vi "Copy Test.vi"() -> ()   [LabVIEW 2020, in "Test Executive.lvlib"]
uses:
  <vilib>/gpm_packages/@cs/test-executive/Source/Test Executive/Test Executive.lvlib
  <vilib>/gpm_packages/@cs/test-executive/Source/Test Executive/TestExecutive/Test Executive.lvclass
  C:/Program Files/National Instruments/LabVIEW 2020/vi.lib/gpm_packages/@cs/test-executive/Source/Test Executive/ITestExecutive/ITest Executive.lvclass
  <vilib>/gpm_packages/@cs/test-executive/Source/Test Executive/Executioner/Executioner.lvclass
  <vilib>/gpm_packages/@cs/run-time-assertions/Source/Assert Equal/Assert Equal.lvclass
  C:/Program Files/National Instruments/LabVIEW 2020/vi.lib/gpm_packages/@cs/run-time-assertions/Source/Assert/Assert.lvclass
  <vilib>/gpm_packages/@cs/run-time-assertions/Source/Assert Greater/Assert Greater.lvclass
  <vilib>/gpm_packages/@cs/run-time-assertions/Source/Assert Less/Assert Less.lvclass
  e1a8998e-4afa-4658-809d-ffab1fdc1dd3.vi
  2b1bbdfa-28ea-4975-b67d-55fb8ecea142.vi
  38d44331-03b6-4e0e-b502-f580cf716a25.vi
  13797e50-8b76-425b-83b2-76a457203fcb.vi
  82e98dc6-0186-4ac9-b806-f29624e46a62.vi
  c7986c9b-765c-4e35-9bdb-656a1762b2cf.vi
  5b298818-1d60-4780-a578-24e6083b1334.vi
  313207bc-dc89-4460-a504-7f065ccd0a73.vi
  3f58f81d-24f4-4b38-8029-ea7739ca710f.vi
  4ea763fe-e262-4f1b-8a79-0ca79b847688.vi
  6a21370e-3cef-4ac3-8829-bf63652873b0.vi
  103630d6-5241-4d15-b3ff-21d61f4a4c4c.vi
  36607b50-8362-4d71-bcc6-c0885ffd9225.vi
  6c5806c5-2cdd-491e-b3b5-fcdc1241d2ce.vi
  b891e3ce-f0ac-467a-8f2d-10a6ff9ae12a.vi
  <vilib>/Utility/error.llb/Error Cluster From Error Code.vi
  <vilib>/gpm_packages/@cs/test-executive/Source/Test Executive/ITestExecutive/ITest Executive.lvclass
  <vilib>/gpm_packages/@cs/test-executive/Source/Test Executive/TestExecutive Ref/TestExecutive Ref.lvclass
panel:
  out "X Var post":string[](array[string])
  out "Y Var post":string[](array[string])
  out "Y Var pre":string[](array[string])
  out "X Var pre":string[](array[string])
  in  "Tree Post Copy":string(tree)
  in  "Tree":string(tree)
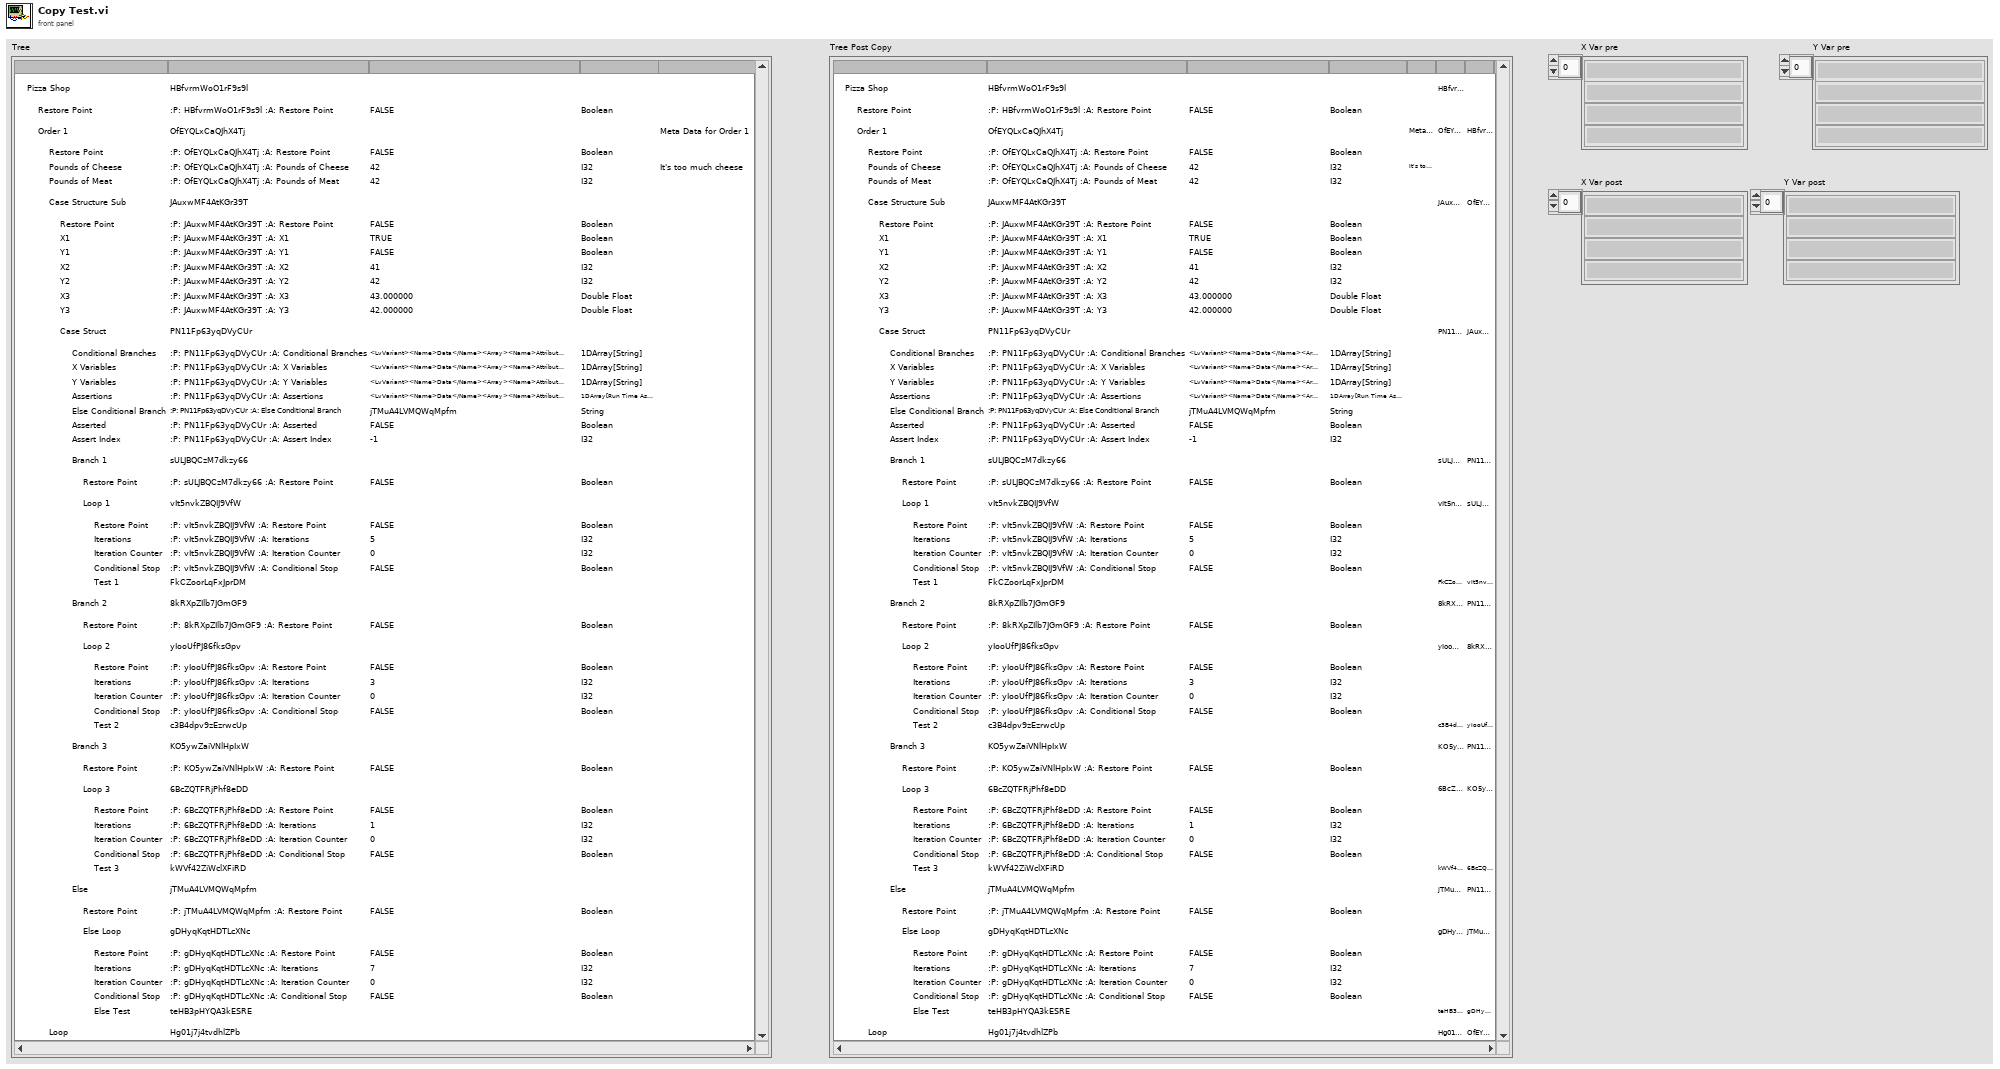
[diagram p1: front panel]
types:
  T1 = cluster{"Left Cell String":string, "Child Text":string[], "Child Tag":string, "Item Indent":i32, "Child Only?":bool, "Glyph Index":i32}[]
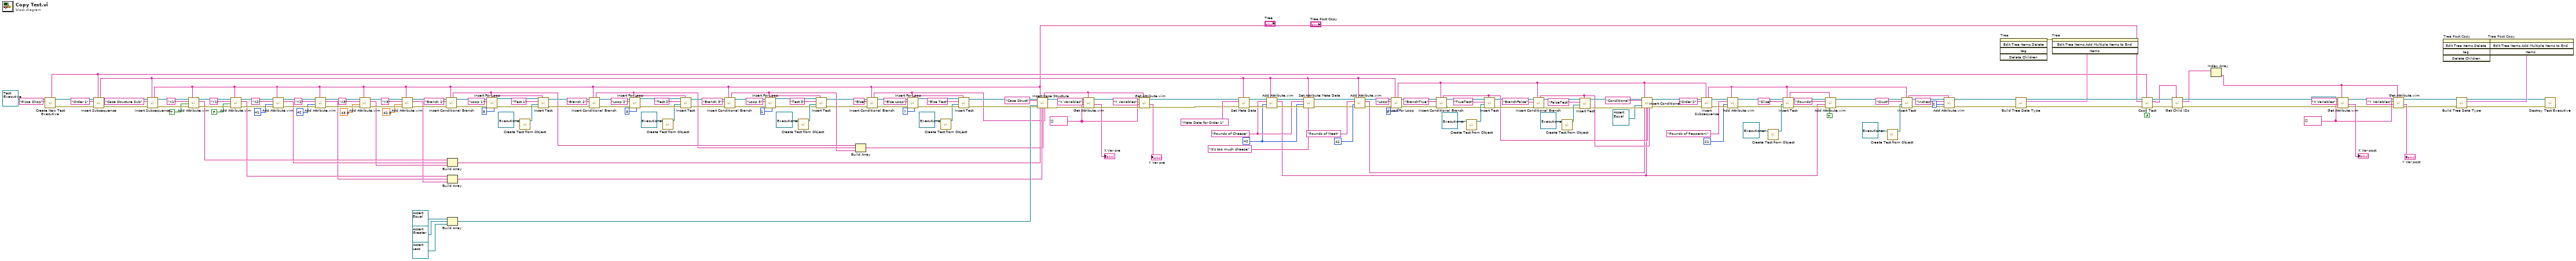
[diagram p0: block diagram]
diagram:
  w15 = string[] []
  w21 = string[] []
  w134 = 42
  w135 = "Pounds of Cheese" ("Attribute Name")
  n1 = call <vilib>:"Create New Test Executive.vi"("Name"="Pizza Shop", "Test Executive"=refnum<class "Test Executive.lvclass"> refnum ("Test Executive.lvlib:Test Executive.lvclass")) -> ("error out"=w208:errorcluster, "Test Executive Ref"=w209:refnum<data-value>, "Test Executive ID out"=w133:string)  [unwired: 7 in]
  n2 = call <vilib>:"Insert Subsequence.vi"("Parent ID"=w133, "error in (no error)"=w208, "Name"="Order 1", "Test Executive Ref"=w209) -> ("error out"=w30:errorcluster, "Test Executive Ref out"=w31:refnum<data-value>, "Unique ID out"=w32:string)  [unwired: 4 in, 1 out]
  n3 = call <vilib>:"Insert Subsequence.vi"("Parent ID"=w32, "error in (no error)"=w30, "Name"="Case Structure Sub", "Test Executive Ref"=w31) -> ("error out"=w127:errorcluster, "Test Executive Ref out"=w128:refnum<data-value>, "Unique ID out"=w8:string)  [unwired: 4 in, 1 out]
  n4 = call "Add Attribute.vim"("ID"=w8, "error in (no error)"=w127, "Attribute"=TRUE, "Attribute Name"="X1", "Test Executive Ref"=w128) -> ("error out"=w121:errorcluster, "Attribute ID out"=w61:string, "Test Executive Ref out"=w122:refnum<data-value>)  [unwired: 3 in, 1 out]
  n5 = call "Add Attribute.vim"("ID"=w8, "error in (no error)"=w121, "Attribute"=FALSE, "Attribute Name"="Y1", "Test Executive Ref"=w122) -> ("error out"=w113:errorcluster, "Attribute ID out"=w58:string, "Test Executive Ref out"=w114:refnum<data-value>)  [unwired: 3 in, 1 out]
  n6 = call "Add Attribute.vim"("ID"=w8, "error in (no error)"=w113, "Attribute"=41, "Attribute Name"="X2", "Test Executive Ref"=w114) -> ("error out"=w120:errorcluster, "Attribute ID out"=w60:string, "Test Executive Ref out"=w119:refnum<data-value>)  [unwired: 3 in, 1 out]
  n7 = call "Add Attribute.vim"("ID"=w8, "error in (no error)"=w120, "Attribute"=42, "Attribute Name"="Y2", "Test Executive Ref"=w119) -> ("error out"=w105:errorcluster, "Attribute ID out"=w57:string, "Test Executive Ref out"=w106:refnum<data-value>)  [unwired: 3 in, 1 out]
  n8 = call "Add Attribute.vim"("ID"=w8, "error in (no error)"=w105, "Attribute"=43.0, "Attribute Name"="X3", "Test Executive Ref"=w106) -> ("error out"=w107:errorcluster, "Attribute ID out"=w59:string, "Test Executive Ref out"=w108:refnum<data-value>)  [unwired: 3 in, 1 out]
  n9 = call "Add Attribute.vim"("ID"=w8, "error in (no error)"=w107, "Attribute"=42.0, "Attribute Name"="Y3", "Test Executive Ref"=w108) -> ("error out"=w102:errorcluster, "Attribute ID out"=w56:string, "Test Executive Ref out"=w104:refnum<data-value>)  [unwired: 3 in, 1 out]
  n10 = call <vilib>:"Insert Conditional Branch.vi"("Parent ID"=w8, "error in (no error)"=w102, "Name"="Branch 1", "Test Executive Ref"=w104) -> ("error out"=w98:errorcluster, "Test Executive Ref out"=w100:refnum<data-value>, "Unique ID out"=w53:string)  [unwired: 4 in, 1 out]
  n11 = Build Array(w61, w60, w59) -> (w55:string[])
  n12 = Build Array(w58, w57, w56) -> (w54:string[])
  n13 = Build Array(refnum<class "Assert Equal.lvclass"> refnum ("Run Time Assertions.lvlib:Assert Equal.lvclass"), refnum<class "Assert Greater.lvclass"> refnum ("Run Time Assertions.lvlib:Assert Greater.lvclass"), refnum<class "Assert Less.lvclass"> refnum ("Run Time Assertions.lvlib:Assert Less.lvclass")) -> (w62:refnum<class "Assert.lvclass">[])
  n14 = call <vilib>:"Insert For Loop.vi"("Loop Iterations"=5, "Parent ID"=w53, "error in (no error)"=w98, "Name"="Loop 1", "Test Executive Ref"=w100) -> ("error out"=w94:errorcluster, "Test Executive Ref out"=w93:refnum<data-value>, "Unique ID out"=w92:string)  [unwired: 3 in, 1 out]
  n15 = call <vilib>:"Create Test from Object.vi"("Test"=refnum<class "Executioner.lvclass"> refnum ("Test Executive.lvlib:Executioner.lvclass")) -> ("Test"=w95:refnum<class "Executioner.lvclass">)  [unwired: 10 in]
  n16 = call <vilib>:"Insert Test.vi"("Parent ID"=w92, "error in (no error)"=w94, "Test"=w95, "Name"="Test 1", "Test Executive Ref"=w93) -> ("error out"=w79:errorcluster, "Test Executive Ref out"=w80:refnum<data-value>)  [unwired: 3 in, 2 out]
  n17 = call <vilib>:"Insert Conditional Branch.vi"("Parent ID"=w8, "error in (no error)"=w79, "Name"="Branch 2", "Test Executive Ref"=w80) -> ("error out"=w85:errorcluster, "Test Executive Ref out"=w83:refnum<data-value>, "Unique ID out"=w52:string)  [unwired: 4 in, 1 out]
  n18 = call <vilib>:"Insert For Loop.vi"("Loop Iterations"=3, "Parent ID"=w52, "error in (no error)"=w85, "Name"="Loop 2", "Test Executive Ref"=w83) -> ("error out"=w89:errorcluster, "Test Executive Ref out"=w90:refnum<data-value>, "Unique ID out"=w91:string)  [unwired: 3 in, 1 out]
  n19 = call <vilib>:"Create Test from Object.vi"("Test"=refnum<class "Executioner.lvclass"> refnum ("Test Executive.lvlib:Executioner.lvclass")) -> ("Test"=w88:refnum<class "Executioner.lvclass">)  [unwired: 10 in]
  n20 = call <vilib>:"Insert Test.vi"("Parent ID"=w91, "error in (no error)"=w89, "Test"=w88, "Name"="Test 2", "Test Executive Ref"=w90) -> ("error out"=w66:errorcluster, "Test Executive Ref out"=w67:refnum<data-value>)  [unwired: 3 in, 2 out]
  n21 = call <vilib>:"Insert Conditional Branch.vi"("Parent ID"=w8, "error in (no error)"=w66, "Name"="Branch 3", "Test Executive Ref"=w67) -> ("error out"=w74:errorcluster, "Test Executive Ref out"=w76:refnum<data-value>, "Unique ID out"=w51:string)  [unwired: 4 in, 1 out]
  n22 = call <vilib>:"Insert For Loop.vi"("Loop Iterations"=1, "Parent ID"=w51, "error in (no error)"=w74, "Name"="Loop 3", "Test Executive Ref"=w76) -> ("error out"=w70:errorcluster, "Test Executive Ref out"=w69:refnum<data-value>, "Unique ID out"=w68:string)  [unwired: 3 in, 1 out]
  n23 = call <vilib>:"Create Test from Object.vi"("Test"=refnum<class "Executioner.lvclass"> refnum ("Test Executive.lvlib:Executioner.lvclass")) -> ("Test"=w71:refnum<class "Executioner.lvclass">)  [unwired: 10 in]
  n24 = call <vilib>:"Insert Test.vi"("Parent ID"=w68, "error in (no error)"=w70, "Test"=w71, "Name"="Test 3", "Test Executive Ref"=w69) -> ("error out"=w37:errorcluster, "Test Executive Ref out"=w38:refnum<data-value>)  [unwired: 3 in, 2 out]
  n25 = Build Array(w53, w52, w51) -> (w50:string[])
  n26 = call <vilib>:"Insert Conditional Branch.vi"("Parent ID"=w8, "error in (no error)"=w37, "Name"="Else", "Test Executive Ref"=w38) -> ("error out"=w43:errorcluster, "Test Executive Ref out"=w41:refnum<data-value>, "Unique ID out"=w34:string)  [unwired: 4 in, 1 out]
  n27 = call <vilib>:"Insert For Loop.vi"("Loop Iterations"=7, "Parent ID"=w34, "error in (no error)"=w43, "Name"="Else Loop", "Test Executive Ref"=w41) -> ("error out"=w47:errorcluster, "Test Executive Ref out"=w48:refnum<data-value>, "Unique ID out"=w49:string)  [unwired: 3 in, 1 out]
  n28 = call <vilib>:"Create Test from Object.vi"("Test"=refnum<class "Executioner.lvclass"> refnum ("Test Executive.lvlib:Executioner.lvclass")) -> ("Test"=w46:refnum<class "Executioner.lvclass">)  [unwired: 10 in]
  n29 = call <vilib>:"Insert Test.vi"("Parent ID"=w49, "error in (no error)"=w47, "Test"=w46, "Name"="Else Test", "Test Executive Ref"=w48) -> ("error out"=w36:errorcluster, "Test Executive Ref out"=w35:refnum<data-value>)  [unwired: 3 in, 2 out]
  n30 = call <vilib>:"Insert Case Structure.vi"("Test Executive Ref"=w35, "Name"="Case Struct", "Assertions"=w62, "error in (no error)"=w36, "Parent ID"=w8, "X Variables"=w55, "Y Variables"=w54, "Conditional Branches"=w50, "\"Else\" Conditional Branch"=w34) -> ("Unique ID out"=w18:string, "Test Executive Ref out"=w29:refnum<data-value>, "error out"=w28:errorcluster)  [unwired: 7 in, 1 out]
  n31 = call "Get Attribute.vim"("ID"=w18, "error in (no error)"=w28, "Type"=w21, "Attribute Name"="X Variables", "Test Executive Ref"=w29) -> ("error out"=w23:errorcluster, "Attribute"=→"X Var pre":string[], "Test Executive Ref out"=w25:refnum<data-value>)  [unwired: 2 in, 2 out]
  n32 = call "Get Attribute.vim"("ID"=w18, "error in (no error)"=w23, "Type"=w21, "Attribute Name"="Y Variables", "Test Executive Ref"=w25) -> ("error out"=w22:errorcluster, "Attribute"=→"Y Var pre":string[], "Test Executive Ref out"=w24:refnum<data-value>)  [unwired: 2 in, 2 out]
  n33 = call <vilib>:"Set Meta Data.vi"("Unique ID"=w32, "error in (no error)"=w22, "Meta Data"="Meta Data for Order 1", "Test Executive Ref"=w24) -> ("error out"=w141:errorcluster, "Test Executive Ref out"=w142:refnum<data-value>)  [unwired: 6 in]
  n34 = call "Add Attribute.vim"("ID"=w32, "error in (no error)"=w141, "Attribute"=w134, "Attribute Name"=w135, "Test Executive Ref"=w142) -> ("error out"=w137:errorcluster, "Attribute ID out"=w130:string, "Test Executive Ref out"=w139:refnum<data-value>)  [unwired: 3 in, 1 out]
  n35 = call <vilib>:"Set Attribute Meta Data.vi"("Meta Data"="It's too much cheese", "Unique ID"=w32, "error in (no error)"=w137, "Attribute Type"=w134, "Attribute Name"=w135, "Test Executive Ref"=w139) -> ("error out"=w136:errorcluster, "Test Executive Ref out"=w138:refnum<data-value>)  [unwired: 3 in, 1 out]
  n36 = call "Add Attribute.vim"("ID"=w32, "error in (no error)"=w136, "Attribute"=42, "Attribute Name"="Pounds of Meat", "Test Executive Ref"=w138) -> ("error out"=w146:errorcluster, "Attribute ID out"=w143:string, "Test Executive Ref out"=w147:refnum<data-value>)  [unwired: 3 in, 1 out]
  n37 = call <vilib>:"Insert For Loop.vi"("Loop Iterations"=5, "Parent ID"=w32, "error in (no error)"=w146, "Name"="Loop", "Test Executive Ref"=w147) -> ("error out"=w152:errorcluster, "Test Executive Ref out"=w154:refnum<data-value>, "Unique ID out"=w150:string)  [unwired: 3 in, 1 out]
  n38 = call <vilib>:"Insert Conditional Branch.vi"("Parent ID"=w150, "error in (no error)"=w152, "Name"="BranchTrue", "Test Executive Ref"=w154) -> ("error out"=w168:errorcluster, "Test Executive Ref out"=w167:refnum<data-value>, "Unique ID out"=w149:string)  [unwired: 4 in, 1 out]
  n39 = call <vilib>:"Create Test from Object.vi"("Test"=refnum<class "Executioner.lvclass"> refnum ("Test Executive.lvlib:Executioner.lvclass")) -> ("Test"=w169:refnum<class "Executioner.lvclass">)  [unwired: 10 in]
  n40 = call <vilib>:"Insert Test.vi"("Parent ID"=w149, "error in (no error)"=w168, "Test"=w169, "Name"="TrueTest", "Test Executive Ref"=w167) -> ("error out"=w161:errorcluster, "Test Executive Ref out"=w160:refnum<data-value>)  [unwired: 3 in, 2 out]
  n41 = call <vilib>:"Insert Conditional Branch.vi"("Parent ID"=w150, "error in (no error)"=w161, "Name"="BranchFalse", "Test Executive Ref"=w160) -> ("error out"=w163:errorcluster, "Test Executive Ref out"=w162:refnum<data-value>, "Unique ID out"=w148:string)  [unwired: 4 in, 1 out]
  n42 = call <vilib>:"Create Test from Object.vi"("Test"=refnum<class "Executioner.lvclass"> refnum ("Test Executive.lvlib:Executioner.lvclass")) -> ("Test"=w164:refnum<class "Executioner.lvclass">)  [unwired: 10 in]
  n43 = call <vilib>:"Insert Test.vi"("Parent ID"=w148, "error in (no error)"=w163, "Test"=w164, "Name"="FalseTest", "Test Executive Ref"=w162) -> ("error out"=w158:errorcluster, "Test Executive Ref out"=w157:refnum<data-value>)  [unwired: 3 in, 2 out]
  n44 = call <vilib>:"Insert Conditional.vi"("Test Executive Ref"=w157, "Name"="Conditional", "Assertion"=refnum<class "Assert Equal.lvclass"> refnum ("Run Time Assertions.lvlib:Assert Equal.lvclass"), "error in (no error)"=w158, "Parent ID"=w150, "Variable X"=w143, "Variable Y"=w130, "Passing Executive"=w149, "Failing Executive"=w148) -> ("Test Executive Ref out"=w153:refnum<data-value>, "error out"=w151:errorcluster)  [unwired: 7 in, 2 out]
  n45 = call <vilib>:"Insert Subsequence.vi"("Parent ID"=w150, "error in (no error)"=w151, "Name"="Order 2", "Test Executive Ref"=w153) -> ("error out"=w206:errorcluster, "Test Executive Ref out"=w205:refnum<data-value>, "Unique ID out"=w174:string)  [unwired: 4 in, 1 out]
  n46 = call "Add Attribute.vim"("ID"=w174, "error in (no error)"=w206, "Attribute"=21, "Attribute Name"="Pounds of Pepperoni", "Test Executive Ref"=w205) -> ("error out"=w193:errorcluster, "Test Executive Ref out"=w194:refnum<data-value>)  [unwired: 3 in, 2 out]
  n47 = call <vilib>:"Create Test from Object.vi"("Test"=refnum<class "Executioner.lvclass"> refnum ("Test Executive.lvlib:Executioner.lvclass")) -> ("Test"=w195:refnum<class "Executioner.lvclass">)  [unwired: 10 in]
  n48 = call <vilib>:"Insert Test.vi"("Parent ID"=w174, "error in (no error)"=w193, "Test"=w195, "Name"="Slice", "Test Executive Ref"=w194) -> ("error out"=w197:errorcluster, "Test Executive Ref out"=w200:refnum<data-value>, "Unique ID out"=w199:string)  [unwired: 3 in, 1 out]
  n49 = call "Add Attribute.vim"("Pointer?"=TRUE, "ID"=w199, "error in (no error)"=w197, "Attribute"=w130, "Attribute Name"="Pounds", "Test Executive Ref"=w200) -> ("error out"=w176:errorcluster, "Test Executive Ref out"=w178:refnum<data-value>)  [unwired: 2 in, 2 out]
  n50 = call <vilib>:"Create Test from Object.vi"("Test"=refnum<class "Executioner.lvclass"> refnum ("Test Executive.lvlib:Executioner.lvclass")) -> ("Test"=w185:refnum<class "Executioner.lvclass">)  [unwired: 10 in]
  n51 = call <vilib>:"Insert Test.vi"("Parent ID"=w174, "error in (no error)"=w176, "Test"=w185, "Name"="Crust", "Test Executive Ref"=w178) -> ("error out"=w183:errorcluster, "Test Executive Ref out"=w180:refnum<data-value>, "Unique ID out"=w173:string)  [unwired: 3 in, 1 out]
  n52 = call "Add Attribute.vim"("ID"=w173, "error in (no error)"=w183, "Attribute"=2, "Attribute Name"="Inches", "Test Executive Ref"=w180) -> ("error out"=w175:errorcluster, "Test Executive Ref out"=w177:refnum<data-value>)  [unwired: 3 in, 2 out]
  n53 = invoke on="Tree" class="Tree (strict)" method="Edit Tree Items.Delete"() -> (error out=w186:errorcluster)  [unwired: 5 in, 4 out]
  n54 = call <vilib>:"Build Tree Data Type.vi"("error in (no error)"=w175, "Test Executive Ref"=w177) -> ("error out"=w188:errorcluster, "Tree Data"=w187:T1, "Test Executive Ref out"=w189:refnum<data-value>)  [unwired: 7 in]
  n55 = invoke on="Tree" class="Tree (strict)" method="Edit Tree Items.Add Multiple Items to End"(error in=w186, "Items"=w187) -> ()  [unwired: 2 in, 4 out]
  n56 = call <vilib>:"Copy Test.vi"("Move?"=FALSE, "New Parent ID"=w133, "error in (no error)"=w188, "Test ID"=w8, "Test Executive Ref"=w189) -> ("error out"=w6:errorcluster, "Test ID out"=w2:string, "Test Executive Ref out"=w7:refnum<data-value>)  [unwired: 4 in]
  n57 = call <vilib>:"Get Child IDs.vi"("Unique ID"=w2, "error in (no error)"=w6, "Test Executive Ref"=w7) -> ("error out"=w4:errorcluster, "Child IDs"=w3:string[], "Test Executive Ref out"=w5:refnum<data-value>)  [unwired: 6 in]
  n58 = Index Array(array=w3) -> (element=w1:string)  [unwired: 1 in]
  n59 = call "Get Attribute.vim"("ID"=w1, "error in (no error)"=w4, "Type"=w15, "Attribute Name"="X Variables", "Test Executive Ref"=w5) -> ("error out"=w14:errorcluster, "Attribute"=→"X Var post":string[], "Test Executive Ref out"=w13:refnum<data-value>)  [unwired: 2 in, 2 out]
  n60 = call "Get Attribute.vim"("ID"=w1, "error in (no error)"=w14, "Type"=w15, "Attribute Name"="Y Variables", "Test Executive Ref"=w13) -> ("error out"=w9:errorcluster, "Attribute"=→"Y Var post":string[], "Test Executive Ref out"=w10:refnum<data-value>)  [unwired: 2 in, 2 out]
  n61 = invoke on="Tree Post Copy" class="Tree (strict)" method="Edit Tree Items.Delete"() -> (error out=w212:errorcluster)  [unwired: 5 in, 4 out]
  n62 = call <vilib>:"Build Tree Data Type.vi"("error in (no error)"=w9, "Test Executive Ref"=w10) -> ("error out"=w210:errorcluster, "Tree Data"=w213:T1, "Test Executive Ref out"=w211:refnum<data-value>)  [unwired: 7 in]
  n63 = invoke on="Tree Post Copy" class="Tree (strict)" method="Edit Tree Items.Add Multiple Items to End"(error in=w212, "Items"=w213) -> ()  [unwired: 2 in, 4 out]
  n64 = call <vilib>:"Destroy Test Executive.vi"("error in (no error)"=w210, "Test Executive Ref"=w211) -> ()  [unwired: 9 in, 1 out]
